vi "WPI_EncoderClose.vi"(8 "error in (no error)":errorcluster, 10 "Close Dependencies":bool=TRUE, 11 "EncoderDevRef":T1={"DevStatus"={"status"=FALSE, "code"=0, "source"=""}, "EncoderIndex"=enum."Invalid", "CounterIndex"=enum."Invalid", "DistancePerCount"=1.0, "Decoding Type"=enum."4x"}) -> (0 "error out":errorcluster)   [LabVIEW 2017]
doc: "Closes the reference to the encoder you specify. Use this VI to close each encoder reference that you open with the Open VI. If you do not stop a running encoder with the Stop VI, closing the reference to the encoder stops the encoder.\n\nThis software is licensed. Open the labview\\readme\\WPI Robotics Library Open Source License.txt file for more information."
uses:
  <vilib>/Rock Robotics/WPI/Encoder/WPI_EncoderDevRef.ctl
  <vilib>/Rock Robotics/SystemInterfaces/Encoder/FPGA_EncoderIdx.ctl
  <vilib>/Rock Robotics/SystemInterfaces/Counter/FPGA_CounterCtrSystemIndex.ctl
  <vilib>/Rock Robotics/WPI/Encoder/WPI_EncoderType.ctl
  <vilib>/Rock Robotics/WPI/Encoder/WPI_EncoderCacheOp.ctl
  <vilib>/Rock Robotics/SystemInterfaces/Encoder/FPGA_EncoderOpen WO Configuration.vi
  <vilib>/Rock Robotics/SystemInterfaces/Encoder/FPGA_EncoderERRInvalidResource.vi
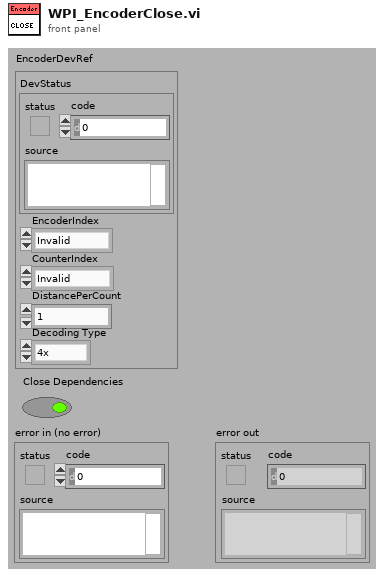
[diagram p1: front panel]
types:
  T1 = typedef "WPI_EncoderDevRef.ctl" = cluster{"DevStatus":errorcluster, "EncoderIndex":T2, "CounterIndex":T3, "DistancePerCount":dbl, "Decoding Type":T4}
  T2 = typedef "FPGA_EncoderIdx.ctl" = enum8{"Enc 0", "Enc 1", "Enc 2", "Enc 3", "Enc 4", "Enc 5", "Enc 6", "Enc 7", "Invalid"}
  T3 = typedef "FPGA_CounterCtrSystemIndex.ctl" = enum8{"Ctr 0", "Ctr 1", "Ctr 2", "Ctr 3", "Ctr 4", "Ctr 5", "Ctr 6", "Ctr 7", "Invalid"}
  T4 = typedef "WPI_EncoderType.ctl" = enum16{"1x", "2x", "4x"}
  T5 = typedef "WPI_EncoderCacheOp.ctl" = enum16{"Acquire", "Release"}
  T6 = typedef "WPI_CounterDevRef.ctl" = cluster{"DevStatus":errorcluster, "CntIndex":T3}
  T7 = typedef "FPGA_EncoderDevRef.ctl" = cluster{"EncoderIndex":T2, "DevStatus":errorcluster}
  T8 = typedef "FPGA_CounterEncoderSourceConvertionLVSourceType.ctl" = cluster{"DevStatus":errorcluster, "AnalogTriggerMode?":bool, "DigitalMode":cluster{"DIO Channel":T9}, "AnalogTriggerMode":cluster{"AnalogTriggerIndex":T10, "OutputType":T11}}
  T9 = typedef "FPGA_DIODigitalSourceChannel.ctl" = enum8{"DIO 0", "DIO 1", "DIO 2", "DIO 3", "DIO 4", "DIO 5", "DIO 6", "DIO 7", "DIO 8", "DIO 9", "DIO MXP 0", "DIO MXP 1", "DIO MXP 2", "DIO MXP 3", "DIO MXP 4", "DIO MXP 5", "DIO MXP 6", "DIO MXP 7", "DIO MXP 8", "DIO MXP 9", "DIO MXP 10", "DIO MXP 11", "DIO MXP 12", "DIO MXP 13", "DIO MXP 14", "DIO MXP 15", "Disabled"}
  T10 = typedef "FPGA_AnalogTriggerIndex.ctl" = enum8{"Trig 0", "Trig 1", "Trig 2", "Trig 3", "Trig 4", "Trig 5", "Trig 6", "Trig 7", "Invalid"}
  T11 = typedef "FPGA_AnalogTriggerOutType.ctl" = enum16{"InWindow", "TriggerState", "Rising", "Falling"}
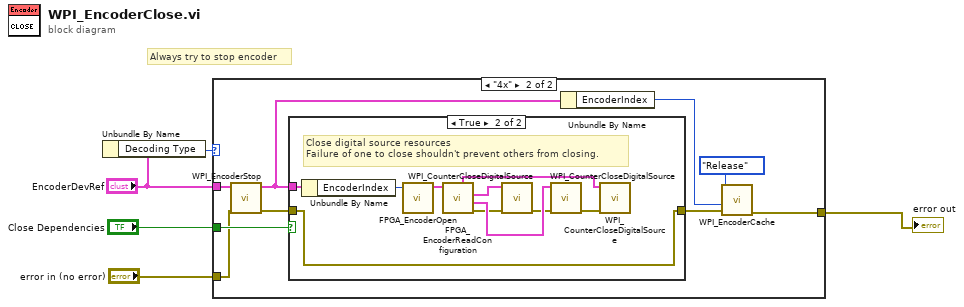
[diagram p0: block diagram]
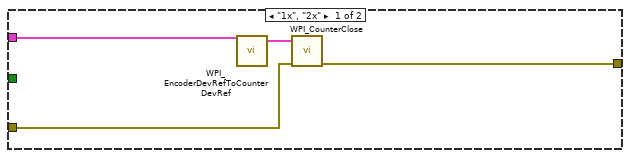
[diagram p2: hidden frame]
diagram:
  # "Always try to stop encoder"
  n1 = Unbundle By Name("EncoderDevRef") -> ("Decoding Type"=w3:T4)
  n2 = case shown="\"4x\"" w3 {
    tunnel: [w7 w11] -> w1
    tunnel: "Close Dependencies" -> [_ w17]
    tunnel: "EncoderDevRef" -> [w9 w13]
    tunnel: "error in (no error)" -> [w6 w10]
    frame "1x", "2x" {
      n3 = call <vilib>:"WPI_EncoderDevRefToCounterDevRef.vi"("EncoderDevRef"=w9) -> ("CounterDevRef"=w8:T6)
      n4 = call <vilib>:"WPI_CounterClose.vi"("error in (no error)"=w6, "CounterDevRef"=w8) -> ("error out"=w7:errorcluster)  [unwired: 1 in, 8 out]
    }
    frame "4x" {
      n5 = call <vilib>:"WPI_EncoderStop.vi"("error in (no error)"=w10, "EncoderDevRef"=w13) -> ("error out"=w15:errorcluster, "EncoderDevRef"=w12:T1)  [unwired: 8 out]
      n6 = case shown="True" w17 {
        tunnel: w12 -> [_ w26]
        tunnel: [w19 w23] -> w16
        tunnel: w15 -> [w19 w23]
        frame False {
        }
        frame True {
          # "Close digital source resources\nFailure of one to close shouldn't prevent others from closing."
          n7 = Unbundle By Name(w26) -> ("EncoderIndex"=w25:T2)
          n8 = call-poly <vilib>:"FPGA_EncoderOpen.vi"("EncoderIndex"=w25) -> ("Encoder Reference"=w24:T7)  [unwired: 2 in, 8 out]
          n9 = call <vilib>:"FPGA_EncoderReadConfiguration.vi"("EncoderDevRef"=w24) -> ("error out"=w22:errorcluster, "BSource"=w28:T8, "ASource"=w29:T8, "IndexSource"=w27:T8)  [unwired: 1 in, 6 out]
          n10 = call <vilib>:"WPI_CounterCloseDigitalSource.vi"("error in"=w22, "UpSource"=w29) -> ("error out"=w20:errorcluster)  [unwired: 5 out]
          n11 = call <vilib>:"WPI_CounterCloseDigitalSource.vi"("error in"=w20, "UpSource"=w28) -> ("error out"=w21:errorcluster)  [unwired: 5 out]
          n12 = call <vilib>:"WPI_CounterCloseDigitalSource.vi"("error in"=w21, "UpSource"=w27) -> ()  [unwired: 6 out]
        }
      }
      n13 = Unbundle By Name(w12) -> ("EncoderIndex"=w14:T2)
      n14 = call <vilib>:"WPI_EncoderCache.vi"("error in (no error)"=w16, "EncoderToRelease"=w14, "Operation"=WPI_EncoderCacheOp."Release") -> ("error out"=w11:errorcluster)  [unwired: 8 out]
    }
  }
  "error out" <- w1
